vi "Send command Get Port.vi"(8 "error in (no error)":errorcluster, 9 "Puerto":string, 10 "Marca":string, 11 "Arduino in":refnum<class "Arduino.lvclass">) -> (0 "error out":errorcluster, 1 "Command":string, 2 "Expected response":string, 3 "Arduino out":refnum<class "Arduino.lvclass">)   [LabVIEW 2020, in "Arduino.lvclass"]
uses:
  Arduino.lvclass
  Arduino.lvclass/Arduino.ctl
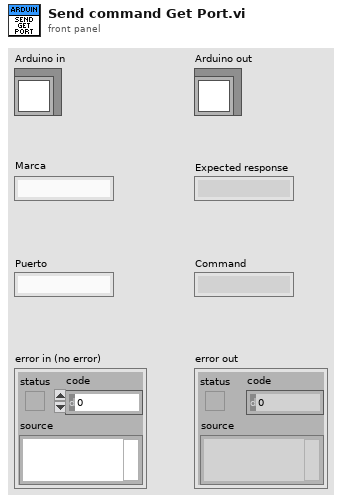
[diagram p1: front panel]
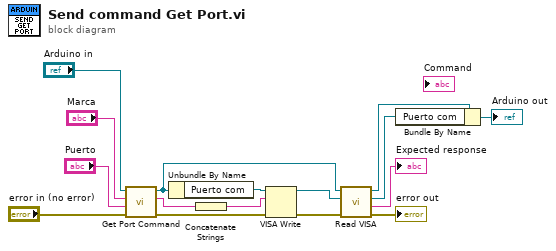
[diagram p0: block diagram]
diagram:
  n1 = call-dynamic "Get Port Command.vi"("error in (no error)"="error in (no error)", "Puerto"="Puerto", "Marca"="Marca", "Serial Device in"="Arduino in") -> ("error out"=w9:errorcluster, "Command"=w8:string, "Serial Device out"=w10:refnum<class "Arduino.lvclass">)  [unwired: 4 in, 1 out]
  n2 = Unbundle By Name(w10) -> ("Puerto com"=w14:refnum<visa-resource-name>)
  n3 = Concatenate Strings(w8) -> (w15:string)
  n4 = VISA Write(VISA resource name=w14, write buffer=w15, error in (no error)=w9) -> (VISA resource name out=w13:refnum<visa-resource-name>, error out=w16:errorcluster)  [unwired: 1 out]
  n5 = call-dynamic "Read VISA.vi"("error in (no error)"=w16, "VISA Refnum in"=w13, "Serial Device in"=w10) -> ("error out"=→"error out":errorcluster, "Serial Response"=→"Expected response":string, "VISA resource name out"=w11:refnum<visa-resource-name>, "Serial Device out"=w12:refnum<class "Arduino.lvclass">)  [unwired: 5 in]
  n6 = Bundle By Name(cluster=w12, "Puerto com"=w11) -> (→"Arduino out":refnum<class "Arduino.lvclass">)
